vi "Get Events.vi"(11 "Test Node Charm View in":refnum<class "Test Node Charm View.lvclass">) -> (2 "Events":T1, 3 "Test Node Charm View out":refnum<class "Test Node Charm View.lvclass">)   [LabVIEW 2013, in "Test Node Charm View.lvlib" / "Test Node Charm View.lvclass"]
uses:
  Test Node Charm View.lvclass
  Typedef/Events.ctl
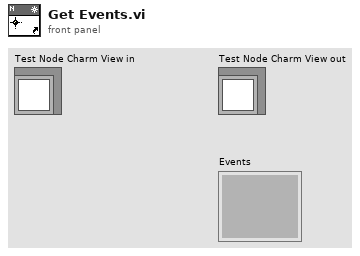
[diagram p1: front panel]
types:
  T1 = typedef "Test Node Charm View.lvlib/Test Node Charm View.lvclass/Events.ctl" = cluster{}
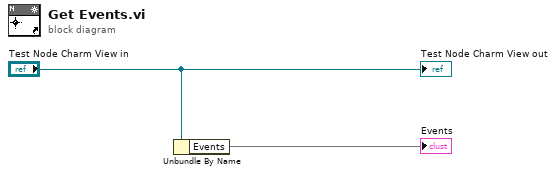
[diagram p0: block diagram]
diagram:
  n1 = Unbundle By Name("Test Node Charm View in") -> ("Events"=→"Events")
  "Test Node Charm View out" <- "Test Node Charm View in"
